vi "CreateControl.vi"(8 "error in (no error)":errorcluster, 11 "BaseAccessorScripter in":refnum<class "BaseAccessorScripter.lvclass">) -> (0 "error out":errorcluster, 2 "New Control Ref":refnum<vi>, 3 "BaseAccessorScripter out":refnum<class "BaseAccessorScripter.lvclass">)   [LabVIEW 2021, in "MemberVICreation.lvlib" / "BaseAccessorScripter.lvclass"]
uses:
  <resource>/Framework/Providers/LVClassLibrary/NewAccessors/BaseAccessorScripter/BaseAccessorScripter.lvclass
  <resource>/Framework/Providers/LVClassLibrary/NewAccessors/BaseAccessorScripter/BaseAccessorScripter.lvclass/BaseAccessorScripter.ctl
  <resource>/Framework/Providers/LVClassLibrary/NewAccessors/MemberVICreation.lvlib
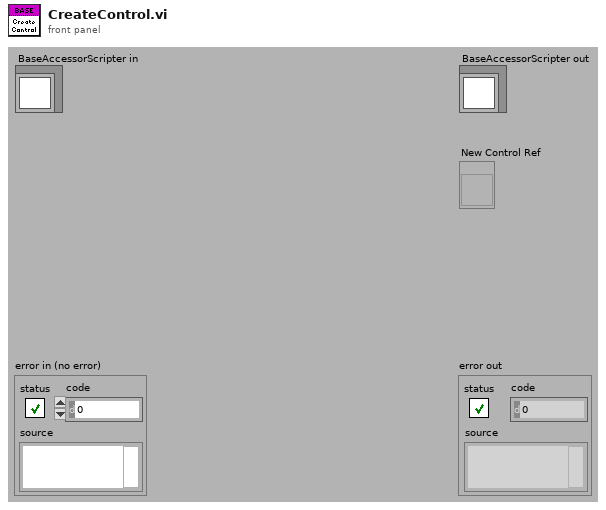
[diagram p1: front panel]
types:
  T1 = enum16{"Invalid Wire Rule", "Required", "Recommended", "Optional", "Dynamic Dispatch"}
  T2 = typedef "LVPositionTypeDef.ctl" = cluster{"Left":i32, "Top":i32}
  T3 = typedef "LVRectTypeDef.ctl" = cluster{"left":i16, "top":i16, "right":i16, "bottom":i16}
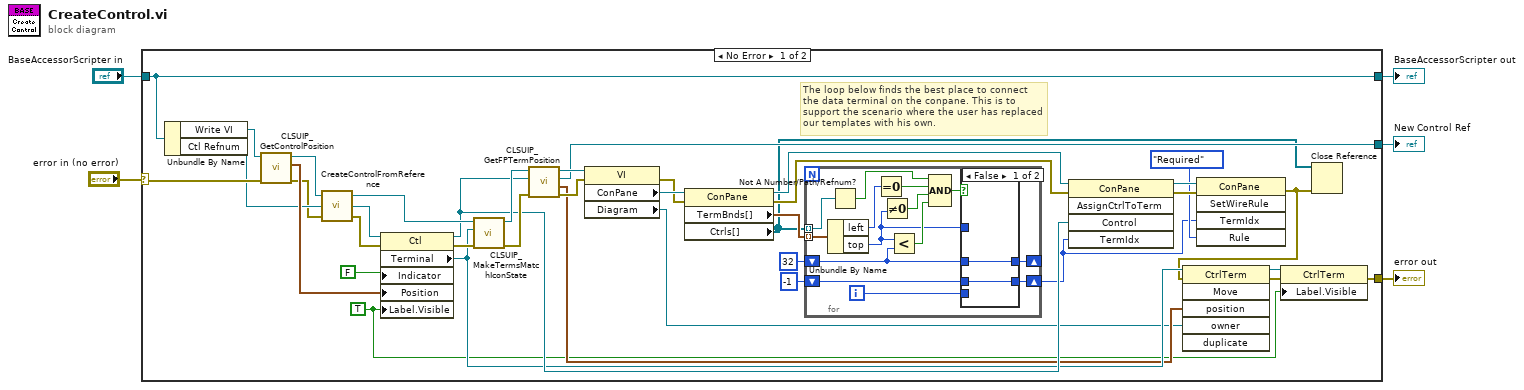
[diagram p0: block diagram]
diagram:
  n1 = case shown="No Error" "error in (no error)" {
    selector: "error in (no error)" -> [w39 w63]
    tunnel: [w32 w63] -> w1
    tunnel: [w42 w62] -> w3
    tunnel: "BaseAccessorScripter in" -> [w42 w62]
    tunnel: [w33 _] -> w2
    frame No Error {
      w8 = TRUE ("Label.Visible")
      # "The loop below finds the best place to connect the data terminal on the conpane. This is to support the scenario where the user has replaced our templates with his own."
      n2 = Unbundle By Name(w42) -> ("Write VI"=w38:refnum<vi>, "Ctl Refnum"=w29:refnum<vi>)
      n3 = call <resource>:"CLSUIP_GetControlPosition.vi"("error in (no error)"=w39, "VI Refnum"=w38) -> ("error out"=w27:errorcluster, "Position"=w37:T2, "VI Refnum out"=w28:refnum<vi>)  [unwired: 7 out]
      n4 = call <resource>:"CreateControlFromReference.vi"("error in (no error)"=w27, "Src CtlRef"=w29, "VI Refnum"=w28) -> ("error out"=w26:errorcluster, "New Object Ref"=w24:refnum<vi>, "VI Refnum out"=w25:refnum<vi>)
      n5 = property class="Ctl"(reference=w24, error in=w26, "Indicator"=FALSE, "Position"=w37, "Label.Visible"=w8) -> (reference out=w20:refnum<vi>, error out=w35:errorcluster, "Terminal"=w19:refnum<vi>)
      n6 = call <resource>:"CLSUIP_MakeTermsMatchIconState.vi"("error in (no error)"=w35, "Terminal"=w19, "VI Refnum"=w25) -> ("error out"=w36:errorcluster, "VI Refnum out"=w34:refnum<vi>)  [unwired: 7 out]
      n7 = call <resource>:"CLSUIP_GetFPTermPosition.vi"("error in (no error)"=w36, "Control Ref"=w20, "VI Refnum"=w34) -> ("error out"=w41:errorcluster, "Position"=w18:cluster{"Left":i32, "Top":i32}, "Control Ref out"=w33:refnum<vi>, "VI Refnum out"=w40:refnum<vi>)  [unwired: 5 out]
      n8 = property class="VI"(reference=w40, error in=w41) -> (error out=w15:errorcluster, "ConPane"=w16:refnum<vi>, "Diagram"=w17:refnum<vi>)  [unwired: 1 out]
      n9 = property class="ConPane"(reference=w16, error in=w15) -> (reference out=w10:refnum<vi>, error out=w11:errorcluster, "TermBnds[]"=w12:T3[], "Ctrls[]"=w6:refnum<vi>[])
      n10 = for {
        tunnel: w12 -> [w47] mode=indexing
        shift-right: [w48] -> _
        shift-left: i16 32 -> [w52]
        shift-right: [w50] -> w9
        shift-left: -1 -> [w51]
        tunnel: w6 -> [w45] mode=indexing
        i -> [w49]
        n11 = Unbundle By Name(w47) -> ("left"=w46:i16, "top"=w53:i16)
        n12 = Not A Number/Path/Refnum?(number/path/refnum=w45) -> (NaN/Path/Refnum?=w44:bool)
        n13 = Equal To 0?(x=w46) -> (x = 0?=w57:bool)
        n14 = Not Equal To 0?(x=w53) -> (x != 0?=w56:bool)
        n15 = Less?(x=w53, y=w52) -> (x < y?=w55:bool)
        n16 = Compound Arithmetic op=AND(w44, w57, w56, w55) -> (w54:bool)
        n17 = case shown="False" w54 {
          tunnel: w53 -> [_ w60]
          tunnel: w52 -> [w59 _]
          tunnel: w51 -> [w58 _]
          tunnel: [w58 w61] -> w50
          tunnel: w49 -> [_ w61]
          tunnel: [w59 w60] -> w48
          frame False {
          }
          frame True {
          }
        }
      }
      n18 = invoke class="ConPane" method="AssignCtrlToTerm"(reference=w10, error in=w11, "Control"=w20, "TermIdx"=w9) -> (reference out=w22:refnum<vi>, error out=w23:errorcluster)  [unwired: 1 in, 3 out]
      n19 = invoke class="ConPane" method="SetWireRule"(reference=w22, error in=w23, "TermIdx"=w9, "Rule"=T1."Required") -> (error out=w7:errorcluster)  [unwired: 1 in, 4 out]
      n20 = invoke class="CtrlTerm" method="Move"(reference=w19, error in=w7, "position"=w18, "owner"=w17) -> (reference out=w30:refnum<vi>, error out=w31:errorcluster)  [unwired: 2 in, 4 out]
      n21 = property class="CtrlTerm"(reference=w30, error in=w31, "Label.Visible"=w8) -> (error out=w32:errorcluster)  [unwired: 1 out]
      n22 = Close Reference(reference=w6, error in (no error)=w7) -> ()  [unwired: 1 out]
    }
    frame Error {
    }
  }
  "error out" <- w1
  "BaseAccessorScripter out" <- w3
  "New Control Ref" <- w2
